vi "输出视图.vi"(8 "error in (no error)":errorcluster caption="错误输入（无错误）", 11 "Nagivation 2.0 输入":refnum<class "Nagivation 2.0.lvclass">) -> (0 "error out":errorcluster caption="错误输出", 3 "Nagivation 2.0 输出":refnum<class "Nagivation 2.0.lvclass">)   [LabVIEW 2018, in "Nagivation 2.0.lvclass"]
uses:
  Nagivation 2.0.lvclass
  <vilib>/picture/cartesn2.llb/XY Plot Type.ctl
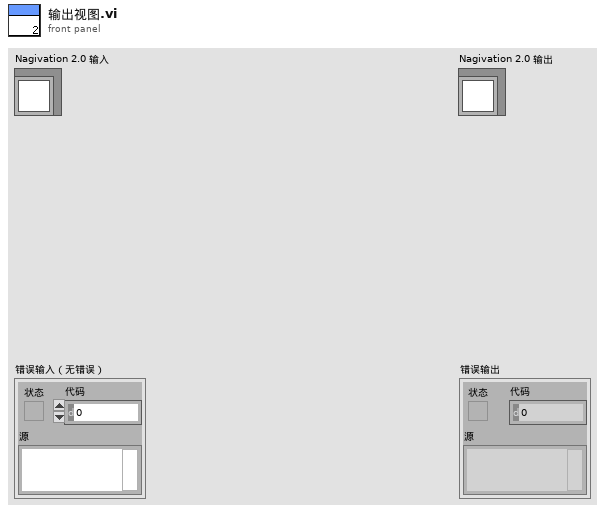
[diagram p1: front panel]
types:
  T1 = typedef "XY Plot Type.ctl" = enum16{"points", "squares", "circles", "connected points", "connected squares", "connected circles", "comb plot", "sized scatter plot", "sized-colored scatter plot", "min-max lines"}
  T2 = cluster{"plot color":u32, "XY plot type":T1, "baseline":dbl}[]
  T3 = cluster{"line color":u32, "text color":u32, "tick length(3)":i16, "crossing axes":bool, "visible grid?":bool}
  T4 = cluster{"x minimum":dbl, "x maximum":dbl, "x log?":bool, "x precision":u8, "x format":enum8{"Decimal", "Scientific", "Engineering", "Binary", "Octal", "Hex"}, "y minimum":dbl, "y maximum":dbl, "y log?":bool, "y precision":u8, "y format":enum8{"Decimal", "Scientific", "Engineering", "Binary", "Octal", "Hex"}}
  T5 = enum16{"User-specified Font", "Application Font", "System Font", "Dialog Font"}
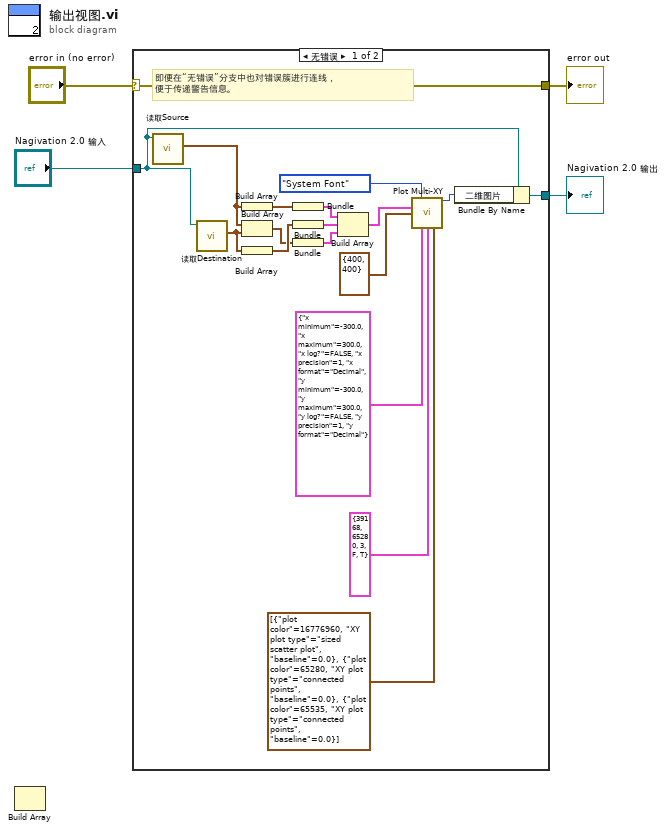
[diagram p0: block diagram]
diagram:
  n1 = Build Array() -> ()  [unwired: 3 in, 1 out]
  n2 = case shown="无错误" "error in (no error)" {
    selector: "error in (no error)" -> [w22 w24]
    tunnel: [w22 w24] -> w3
    tunnel: [w5 w23] -> w1
    tunnel: "Nagivation 2.0 输入" -> [w12 w23]
    frame No Error {
      # "即便在“无错误”分支中也对错误簇进行连线，\n便于传递警告信息。"
      n3 = call-dynamic "读取Source.vi"("Navigation输入"=w12) -> ("Source"=w9:cluster{"X":dbl, "Y":dbl})  [unwired: 8 in, 2 out]
      n4 = call-dynamic "读取Destination.vi"("Navigation输入"=w12) -> ("Destination"=w8:cluster{"X":dbl, "Y":dbl})  [unwired: 8 in, 2 out]
      n5 = Build Array(w9) -> (w15:cluster{"X":dbl, "Y":dbl}[])
      n6 = Build Array(w9, w8) -> (w7:cluster{"X":dbl, "Y":dbl}[])
      n7 = Build Array(w8) -> (w11:cluster{"X":dbl, "Y":dbl}[])
      n8 = Bundle(w15) -> (w14:cluster{cluster{"X":dbl, "Y":dbl}[]})  [unwired: 1 in]
      n9 = Bundle(w11) -> (w10:cluster{cluster{"X":dbl, "Y":dbl}[]})  [unwired: 1 in]
      n10 = Bundle(w7) -> (w6:cluster{cluster{"X":dbl, "Y":dbl}[]})  [unwired: 1 in]
      n11 = Build Array(w14, w10, w6) -> (w13:cluster{cluster{"X":dbl, "Y":dbl}[]}[])
      n12 = call <vilib>:"Plot Multi-XY.vi"("desired font(Application)"=T5."System Font", "data"=w13, "dimensions (w,h)"=cluster{"width":i16, "height":i16} {"width"=400, "height"=400}, "cartesian axis attributes"=T4 {"x minimum"=-300.0, "x maximum"=300.0, "x log?"=FALSE, "x precision"=1, "x format"=enum."Decimal", "y minimum"=-300.0, "y maximum"=300.0, "y log?"=FALSE, "y precision"=1, "y format"=enum."Decimal"}, "cartesian grid cosmetics"=T3 {"line color"=39168, "text color"=65280, "tick length(3)"=3, "crossing axes"=FALSE, "visible grid?"=TRUE}, "XY plot cosmetics"=T2 [{"plot color"=16776960, "XY plot type"=enum."sized scatter plot", "baseline"=0.0}, {"plot color"=65280, "XY plot type"=enum."connected points", "baseline"=0.0}, {"plot color"=65535, "XY plot type"=enum."connected points", "baseline"=0.0}]) -> ("new picture"=w16:picture)  [unwired: 9 in]
      n13 = Bundle By Name(cluster=w12, "二维图片"=w16) -> (w5:refnum<class "Nagivation 2.0.lvclass">)
    }
    frame Error {
    }
  }
  "error out" <- w3
  "Nagivation 2.0 输出" <- w1
